vi "Remove Task Request.vi"(8 "error in (no error)":errorcluster, 10 "Task":variant, 11 "BuildWorker in":refnum<class "BuildWorker.lvclass">) -> (0 "error out":errorcluster, 3 "BuildWorker out":refnum<class "BuildWorker.lvclass">)   [LabVIEW 2017, in "BuildWorker.lvlib" / "BuildWorker.lvclass"]
uses:
  BuildWorker.lvclass
  Classes/Task/Task.lvclass
  Classes/Task/Status.ctl
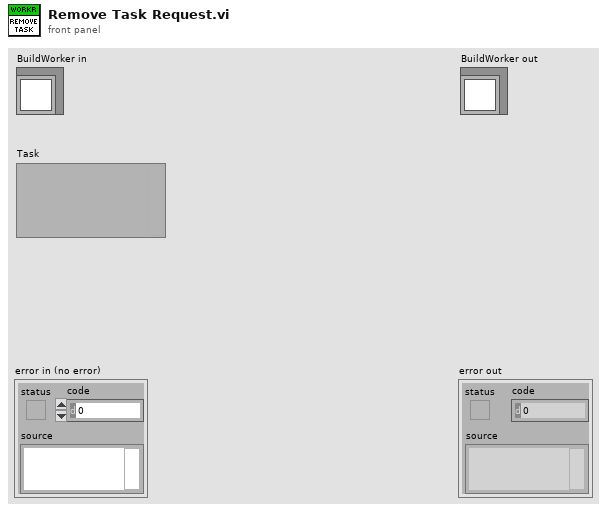
[diagram p1: front panel]
types:
  T1 = typedef "Task Interface.lvlib/Task.lvclass/Status.ctl" = enum16{"Created", "Added", "Pending", "Queued", "Processing", "Cleaning", "Building", "Finished", "Failed", "Removed", "Not found"}
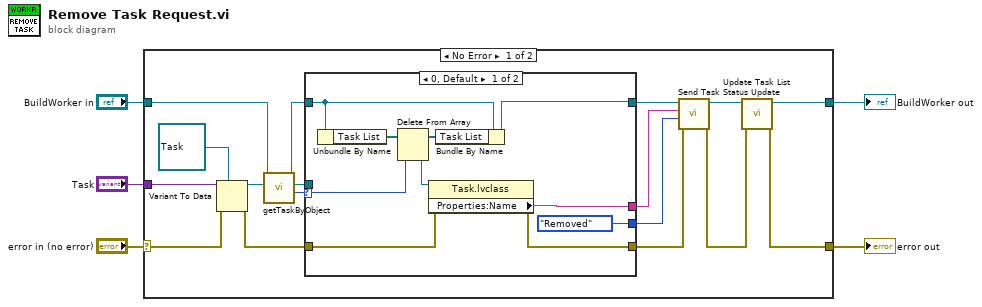
[diagram p0: block diagram]
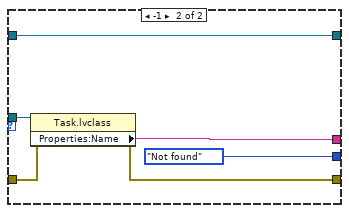
[diagram p2: hidden frame]
diagram:
  n1 = case shown="No Error" "error in (no error)" {
    selector: "error in (no error)" -> [w20 w40]
    tunnel: [w17 w40] -> w4
    tunnel: [w18 w39] -> w2
    tunnel: "BuildWorker in" -> [w16 w39]
    tunnel: "Task" -> [w22 _]
    frame No Error {
      n2 = Variant To Data(error in=w20, type=refnum<class "Task.lvclass"> refnum ("Task.lvclass"), Variant=w22) -> (data=w15:refnum<class "Task.lvclass">, error out=w19:errorcluster)
      n3 = call "getTaskByObject.vi"("Task Object"=w15, "BuildWorker in"=w16) -> ("index of element"=w14:i32, "Task"=w13:refnum<class "Task.lvclass">, "BuildWorker out"=w12:refnum<class "BuildWorker.lvclass">)  [unwired: 7 in]
      n4 = case shown="0, Default" w14 {
        selector: w14 -> [w32 _]
        tunnel: [w30 w34] -> w7
        tunnel: w19 -> [w31 w35]
        tunnel: w13 -> [_ w38]
        tunnel: [w29 w37] -> w9
        tunnel: w12 -> [w27 w36]
        tunnel: [w26 w36] -> w11
        tunnel: [Status."Removed" ("Status") Status."Not found" ("Status")] -> w8
        frame 0, Default {
          n5 = Unbundle By Name(w27) -> ("Task List"=w28:refnum<class "Task.lvclass">[])
          n6 = Delete From Array(array=w28, index=w32) -> (deleted portion=w24:refnum<class "Task.lvclass">, array with subset deleted=w25:refnum<class "Task.lvclass">[])  [unwired: 1 in]
          n7 = property class="Task.lvclass"(reference=w24, error in=w31) -> (error out=w30:errorcluster, "Properties:Name"=w29:string)  [unwired: 1 out]
          n8 = Bundle By Name(cluster=w27, "Task List"=w25) -> (w26:refnum<class "BuildWorker.lvclass">)
        }
        frame -1 {
          n9 = property class="Task.lvclass"(reference=w38, error in=w35) -> (error out=w34:errorcluster, "Properties:Name"=w37:string)  [unwired: 1 out]
        }
      }
      n10 = call "Send Task Status Update.vi"("error in (no error)"=w7, "Status"=w8, "Task Name"=w9, "BuildWorker in"=w11) -> ("error out"=w6:errorcluster, "BuildWorker out"=w10:refnum<class "BuildWorker.lvclass">)  [unwired: 6 in]
      n11 = call "Update Task List.vi"("error in (no error)"=w6, "BuildWorker in"=w10) -> ("error out"=w17:errorcluster, "BuildWorker out"=w18:refnum<class "BuildWorker.lvclass">)  [unwired: 8 in]
    }
    frame Error {
    }
  }
  "error out" <- w4
  "BuildWorker out" <- w2
